vi "Check IR Breakbeam.vi"() -> (0 "Beam Broken":bool)   [LabVIEW 2015]
uses:
  Robot Global Data.vi
panel:
  in  "Beam Broken":bool
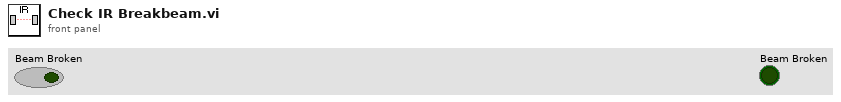
[diagram p1: front panel]
types:
  T1 = typedef "WPI_DigitalInputDevRef.ctl" = cluster{"DevStatus":errorcluster, "DIO Channel":T2}
  T2 = typedef "FPGA_DIOChannel.ctl" = enum8{"DIO 0", "DIO 1", "DIO 2", "DIO 3", "DIO 4", "DIO 5", "DIO 6", "DIO 7", "DIO 8", "DIO 9", "DIO MXP 0", "DIO MXP 1", "DIO MXP 2", "DIO MXP 3", "DIO MXP 4", "DIO MXP 5", "DIO MXP 6", "DIO MXP 7", "DIO MXP 8", "DIO MXP 9", "DIO MXP 10", "DIO MXP 11", "DIO MXP 12", "DIO MXP 13", "DIO MXP 14", "DIO MXP 15", "Invalid"}
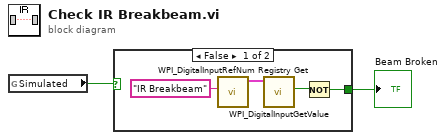
[diagram p0: block diagram]
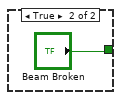
[diagram p2: hidden frame]
diagram:
  n1 = global read "Robot Global Data.vi" "Simulated"() -> (w1:bool)
  n2 = case shown="False" w1 {
    tunnel: [w5 "Beam Broken"] -> w2
    frame False {
      n3 = call <vilib>:"WPI_DigitalInputRefNum Registry Get.vi"("refnum name"="IR Breakbeam") -> ("DigitalInputDevRef"=w3:T1)  [unwired: 9 in, 1 out]
      n4 = call <vilib>:"WPI_DigitalInputGetValue.vi"("DigitalInputDevRef"=w3) -> ("Value"=w6:bool)  [unwired: 8 in, 2 out]
      n5 = Not(x=w6) -> (.not. x?=w5:bool)
    }
    frame True {
    }
  }
  "Beam Broken" <- w2
